vi "Read First phase word.vi"(8 "error in (no error)":errorcluster, 11 "RP Transceiver in":refnum<class "RP Transceiver.lvclass">) -> (0 "error out":errorcluster, 2 "First phase word":i32, 3 "RP Transceiver out":refnum<class "RP Transceiver.lvclass">)   [LabVIEW 2024, in "RP Transceiver.lvclass"]
uses:
  RP Transceiver.lvclass
  RP Transceiver.lvclass/RP Transceiver.ctl
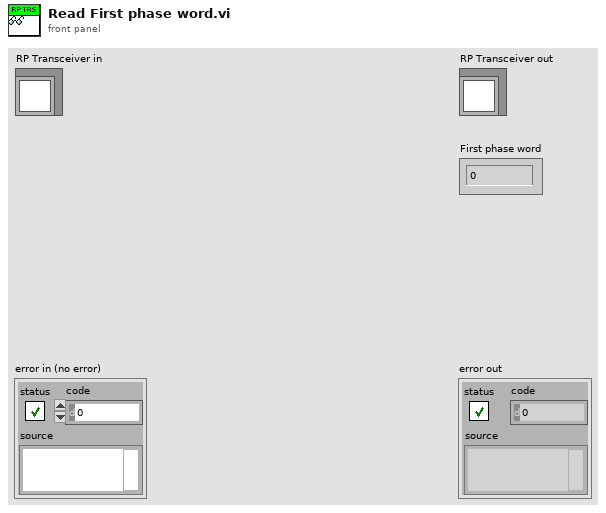
[diagram p1: front panel]
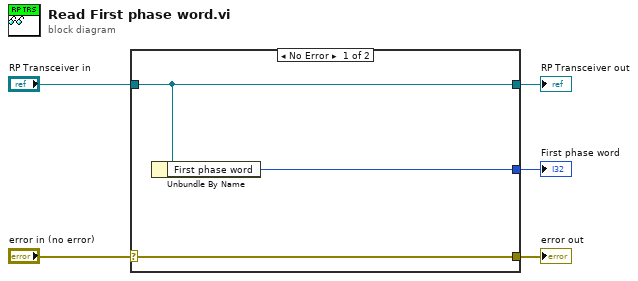
[diagram p0: block diagram]
diagram:
  n1 = case shown="No Error" "error in (no error)" {
    selector: "error in (no error)" -> [w8 w9]
    tunnel: [w8 w9] -> w4
    tunnel: [w7 w10] -> w2
    tunnel: "RP Transceiver in" -> [w7 w10]
    tunnel: [w6 _] -> w1
    frame No Error {
      n2 = Unbundle By Name(w7) -> ("First phase word"=w6:i32)
    }
    frame Error {
    }
  }
  "error out" <- w4
  "RP Transceiver out" <- w2
  "First phase word" <- w1
